vi "ADV VEL PID 3.vi"(9 "Time":dbl, 10 "SP-SetPoint":dbl=-0.0, 11 "PV-Measurement":dbl=2.126342861032265e-06) -> (3 "CO-ControlOutput":dbl=-2.828036005172913e-07)   [LabVIEW 2020]
uses:
  <vilib>/Rock Robotics/WPI/ThirdParty/JAS_Junk/TrajLib/PIDController_AtSetpoint.vi
  <vilib>/Rock Robotics/WPI/ThirdParty/JAS_Junk/TrajLib/PIDController_SetPIDF.vi
  <vilib>/Rock Robotics/WPI/ThirdParty/JAS_Junk/TrajLib/PIDController_SetDerivativeFilter.vi
  <vilib>/Rock Robotics/WPI/ThirdParty/JAS_Junk/TrajLib/PIDController_SetIntegratorRange.vi
  <vilib>/Rock Robotics/WPI/ThirdParty/JAS_Junk/TrajLib/PIDController_SetTolerancePandV.vi
  <vilib>/Rock Robotics/WPI/ThirdParty/JAS_Junk/TrajLib/PIDController_DisableContinousInput.vi
  <vilib>/Rock Robotics/WPI/ThirdParty/JAS_Junk/TrajLib/PIDController_EnableContinousInput.vi
  <vilib>/Rock Robotics/WPI/ThirdParty/JAS_Junk/TrajLib/PIDController_Reset.vi
  <vilib>/Rock Robotics/WPI/ThirdParty/JAS_Junk/TrajLib/PIDController_New.vi
  <vilib>/Rock Robotics/WPI/ThirdParty/JAS_Junk/TrajLib/PIDController_SetOutputLimits.vi
  <vilib>/Rock Robotics/WPI/ThirdParty/JAS_Junk/TrajLib/PIDController_NewPeriod.vi
  <vilib>/Rock Robotics/SystemInterfaces/NetworkCommunication/NetComm_UsageReport_report.vi
  <vilib>/Rock Robotics/WPI/ThirdParty/JAS_Junk/TrajLib/Globals/Util_LibraryGlobals.vi
  <vilib>/Rock Robotics/WPI/ThirdParty/JAS_Junk/TrajLib/PIDController_AdvCalculate_FF_Sp_Pv.vi
  <vilib>/Rock Robotics/WPI/ThirdParty/JAS_Junk/TrajLib/Trajectory_Library.lvlib
panel:
  in  "Kd":dbl=-0.0 format="%#_13g"
  in  "Ki":dbl format="%#_13g"
  in  "Kp":dbl=0.133 format="%#_13g"
  in  "Kf":dbl=0.4 format="%#_13g"
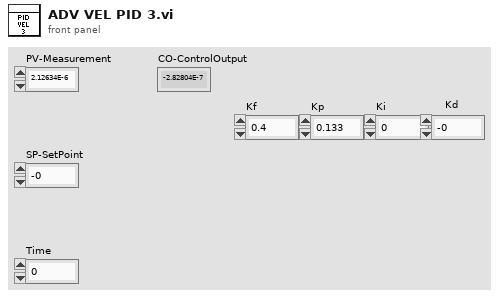
[diagram p1: front panel]
types:
  T1 = typedef "Trajectory_Library.lvlib/PID_ADV_LIMITS.ctl" = cluster{"MaxInput":dbl, "MinInput":dbl, "Continuous":bool, "MaxOutput":dbl, "MinOutput":dbl}
  T2 = typedef "Trajectory_Library.lvlib/PID_ADV_TUNING.ctl" = cluster{"Kf":dbl, "Kp":dbl, "Ki":dbl, "Kd":dbl, "MaximumIntegral":dbl, "MinimumIntegral":dbl, "Filter Derivative":bool}
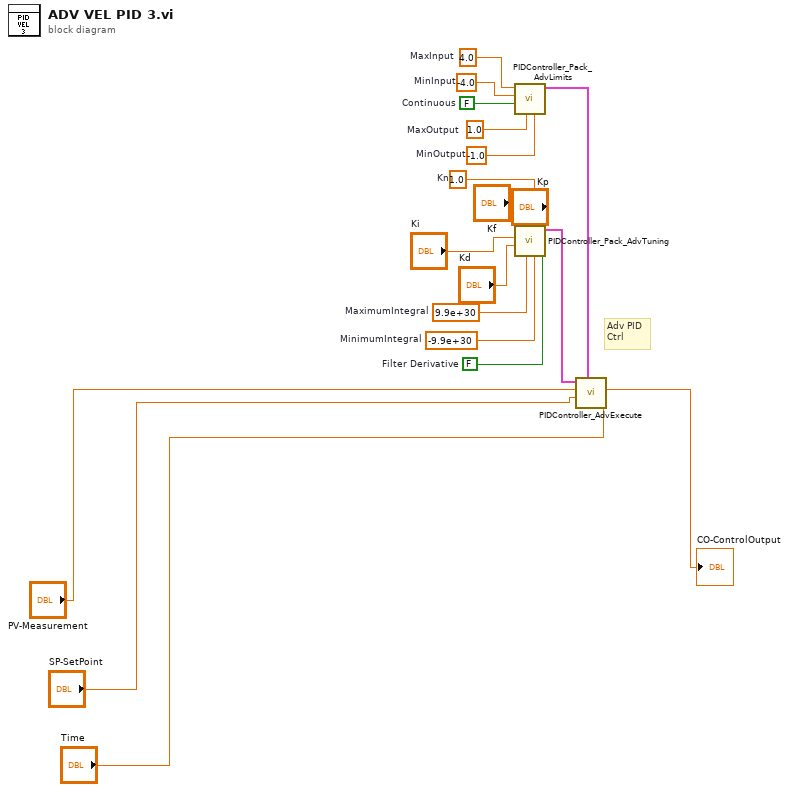
[diagram p0: block diagram]
diagram:
  w1 = 1.0  # Kn
  w6 = 9.9e+30  # MaximumIntegral
  w7 = -9.9e+30  # MinimumIntegral
  w8 = FALSE  # Filter Derivative
  w10 = -4.0  # MinInput
  w11 = FALSE  # Continuous
  w12 = 1.0  # MaxOutput
  w9 = -1.0  # MinOutput
  w13 = 4.0  # MaxInput
  # "Adv PID\nCtrl"
  n1 = call <vilib>:"PIDController_Pack_AdvLimits.vi"("MinOutput"=w9, "MaxOutput"=w12, "Continuous"=w11, "MinInput"=w10, "MaxInput"=w13) -> ("Adv PID Limits"=w15:T1)  [unwired: 6 in]
  n2 = call <vilib>:"PIDController_Pack_AdvTuning.vi"("Filter Derivative"=w8, "MinimumIntegral"=w7, "Kn"=w1, "MaximumIntegral"=w6, "Kf"="Kf", "Kd"="Kd", "Ki"="Ki", "Kp"="Kp") -> ("Adv PID Tuning"=w14:T2)  [unwired: 3 in]
  n3 = call <vilib>:"PIDController_AdvExecute.vi"("Time"="Time", "Adv PID Limits"=w15, "SP-SetPoint"="SP-SetPoint", "PV-Measurement"="PV-Measurement", "Adv PID Tuning"=w14) -> ("CO-ControlOutput"=→"CO-ControlOutput":dbl)  [unwired: 4 in, 2 out]
